vi "Send Error Report.vi"(8 "error in (no error)":errorcluster, 9 "Message Priority (Normal)":T1=enum."Normal", 10 "Error From Sender":errorcluster, 11 "Message Enqueuer":refnum<class "Message Enqueuer.lvclass">) -> (0 "error out":errorcluster)   [LabVIEW 2020, in "Actor Framework.lvlib" / "Report Error Msg.lvclass"]
doc: "<p>(<strong>Filename</strong>: <span class=\"dnl\">Actor Framework.lvlib:Report Error Msg.lvclass:Send Error Report.vi</span>)</p>\n\n<p>Use this VI to send an error to an actor. The error will be handled by the Handle Error VI of the actor. If the error is not handled there, it will cause the actor to stop running.</p>"
uses:
  Report Error Msg.lvclass
  Report Error Msg.lvclass/Report Error Msg.ctl
  Message Enqueuer/Message Enqueuer.lvclass
  C:/justACS/Actor Framework/Core/ActorFramework/Message/Message.lvclass
  C:/justACS/Actor Framework/Core/ActorFramework/Specialty Messages/Report Error Msg/Report Error Msg.lvclass
  Message Enqueuer/Message Priority.ctl
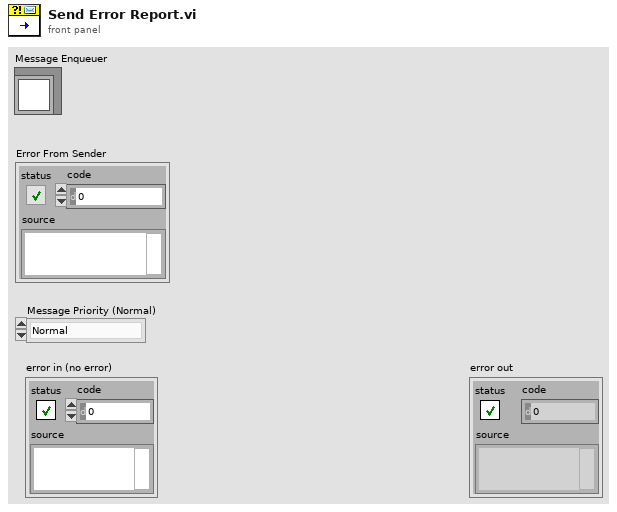
[diagram p1: front panel]
types:
  T1 = typedef "Actor Framework.lvlib/Message Enqueuer.lvclass/Message Priority.ctl" = enum16{"Low", "Normal", "High"}
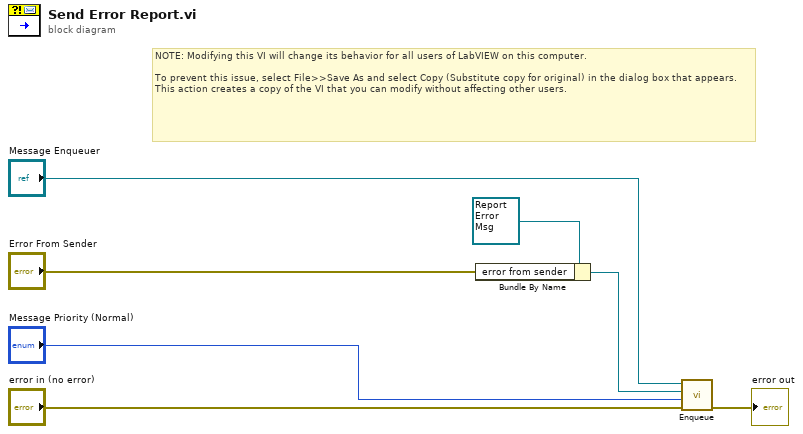
[diagram p0: block diagram]
diagram:
  # "NOTE: Modifying this VI will change its behavior for all users of LabVIEW on this computer.\n\nTo prevent this issue, select File>>Save As and select Copy (Substitute copy for original) in the dialog box that appears. This action creates a copy of the VI that you can modify without affecting other users."
  n1 = Bundle By Name(cluster=refnum<class "Report Error Msg.lvclass"> refnum ("Report Error Msg in"), "error from sender"="Error From Sender") -> (w2:refnum<class "Report Error Msg.lvclass">)
  n2 = call "Enqueue.vi"("error in (no error)"="error in (no error)", "Message Priority (Normal)"="Message Priority (Normal)", "Message"=w2, "Message Enqueuer in"="Message Enqueuer") -> ("error out"=→"error out":errorcluster)  [unwired: 6 in, 1 out]
